vi "xy file read.vi"(9 "#Pins":u8, 10 "Data Array":dbl[][](array[numeric]), 11 "X-Axis Array":dbl[][](array[numeric])) -> (2 "Data Array output":dbl[][](array[numeric]), 3 "X-Axis Array output":dbl[][](array[numeric]))   [LabVIEW 2019]
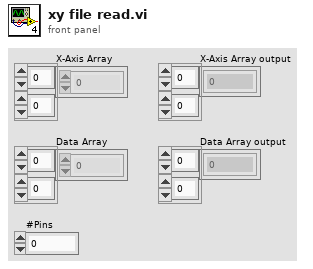
[diagram p1: front panel]
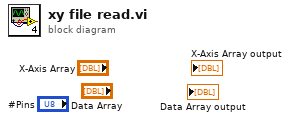
[diagram p0: block diagram]
diagram:
